vi "7-1.vi"() -> ()   [LabVIEW 2017]
panel:
  in  "Knob":dbl(knob) scale=0.0..100.0
  out "Slide":dbl(slide) scale=0.0..100.0
  in  "Stop Button":bool
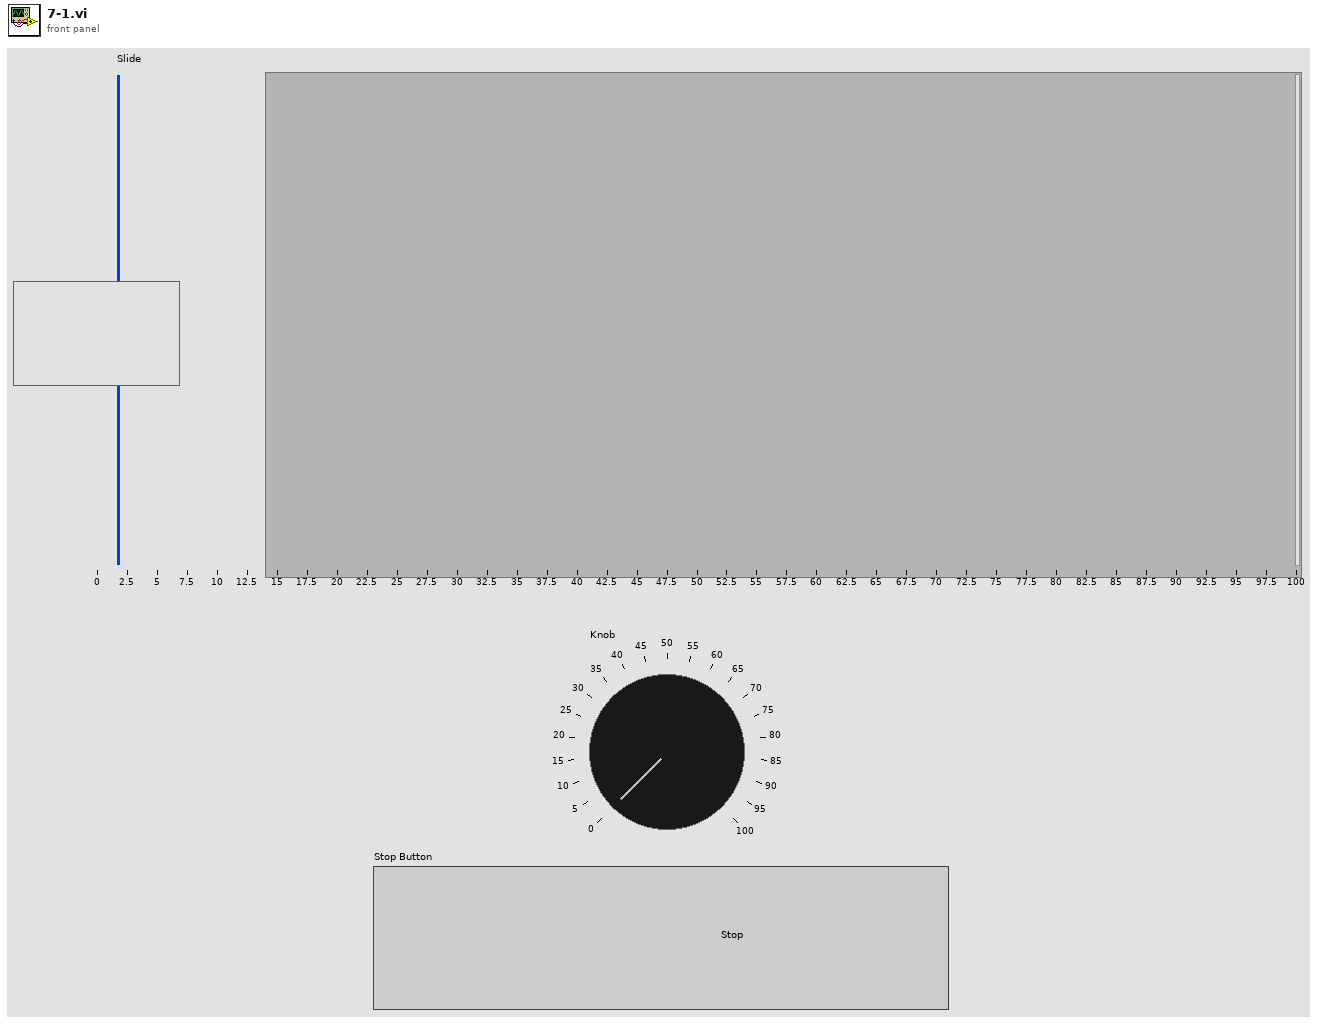
[diagram p1: front panel]
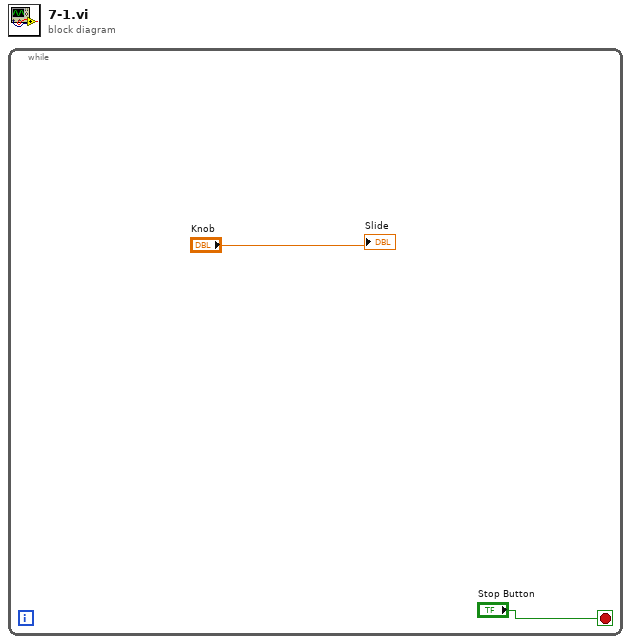
[diagram p0: block diagram]
diagram:
  n1 = while {
    stop <- "Stop Button" stop-if-true
    "Slide" <- "Knob"
  }
